vi "HFRR ADV v030 new software.vi"() -> ()   [LabVIEW 2025] (continued)
          frame #2 {
            n1890 = disable-structure shown="Disabled" {
              frame Disabled {
                w2654 = "cmd.exe  /c \"C:\\LAB-IQ-NXT\\UNOCOMPILE.bat\"" ("string")
                n1891 = local write "Prog Uno"(FALSE ("run minimized? (F)")) -> ()
                n1892 = call <vilib>:"System Exec.vi"("expected output size  (4096)"=u32 65535, "run minimized? (F)"=FALSE, "wait until completion? (T)"=TRUE ("run minimized? (F)"), "working directory"=path "C:/LAB-IQ-NXT", "standard input"=w2654, "command line"=w2654) -> ("error out"=w2653:errorcluster, "standard output"=→"String 42":string)  [unwired: 2 in, 2 out]
                "error out 3" <- w2653
                n1893 = flat-sequence {
                  tunnel: w2653 -> [_]
                  frame #0 {
                  }
                }
              }
              frame Enabled {
              }
            }
          }
        }
      }
    }
    n1894 = case shown="\"ISO 12156\"" "TEST STANDARD" {
      frame "ASTM D6079", Default {
        w2623 = 50.0 ("Hz")
        w2624 = 53.0 ("Set Rh")
        w2626 = 1.0 ("Set Strk")
        w2625 = 60.0 ("Set Temp")
        # "astm hide"
        n1895 = local write "NORMAL LOAD"(200.0 ("NORMAL LOAD")) -> ()
        n1896 = local write "Set Strk"(w2626) -> ()
        n1897 = local write "Set Hz"(w2623) -> ()
        n1898 = local write "Set Temp"(w2625) -> ()
        n1899 = local write "Set Rh"(w2624) -> ()
        n1900 = local write "test time"(75.0 ("test time")) -> ()
        n1901 = local write "Set Stroke:"(w2626) -> ()
        n1902 = local write "Set Humidity:"(w2624) -> ()
        n1903 = local write "Set Frequency:"(w2623) -> ()
        n1904 = local write "Set Temperature:"(w2625) -> ()
        "Test Standard" <- "ASTM D6079" ("Test Standard 2")
      }
      frame "ISO 12156" {
        n1905 = local write "Set Strk"(1.0 ("Set Strk")) -> ()
        n1906 = local write "NORMAL LOAD"(200.0 ("NORMAL LOAD")) -> ()
        n1907 = local write "Set Temp"(60.0 ("Set Temp")) -> ()
        n1908 = local write "test time"(75.0 ("test time")) -> ()
        n1909 = local write "Set Hz"(50.0 ("Hz")) -> ()
        n1910 = local write "Set Rh"(53.0 ("Set Rh")) -> ()
      }
      frame "CEC F-096-A-06" {
        n1911 = local write "Set Strk"(1.0 ("Set Strk")) -> ()
        n1912 = local write "NORMAL LOAD"(200.0 ("NORMAL LOAD")) -> ()
        n1913 = local write "Set Temp"(60.0 ("Set Temp")) -> ()
        n1914 = local write "test time"(75.0 ("test time")) -> ()
        n1915 = local write "Set Hz"(50.0 ("Hz")) -> ()
        n1916 = local write "Set Rh"(53.0 ("Set Rh")) -> ()
      }
      frame "Custom" {
      }
    }
    n1917 = Or(x=w2176, y=w2174) -> (x .or. y?=w2175:bool)
    n1918 = case shown="\"About\"" w2173 {
      tunnel: [T27."Acquire" ("Main Tab") T27."Compare Files" ("Main Tab") T27."About" ("Main Tab")] -> w2184
      frame "Acquire", Default {
      }
      frame "Compare Files" {
      }
      frame "About" {
      }
    }
    n1919 = Or(x=w2179, y="OPEN") -> (x .or. y?=w2180:bool)
    n1920 = case shown="True" w2180 {
      tunnel: w2179 -> [_ w2212]
      frame False {
      }
      frame True {
        n1921 = stacked-sequence {
          tunnel: w2212 -> [_ w2279 _ _]
          frame #0 {
            w2228 = "  " ("String 6")
            n1922 = local write "OPEN"(FALSE ("open")) -> ()
            n1923 = local read "string1 2"() -> (w2216:string)
            n1924 = local read "string1 3"() -> (w2215:string)
            n1925 = local read "string1 4"() -> (w2214:string)
            n1926 = property on="OPEN" class="Bool (strict)"("Visible"=FALSE) -> ()  [unwired: 2 in, 2 out]
            n1927 = local write "String 6"(w2228) -> ()
            n1928 = local write "String 7"(w2228) -> ()
            n1929 = local write "String 8"(w2228) -> ()
            n1930 = local write "String 12"(w2228) -> ()
            n1931 = local read "OK Button 16"() -> (w2213:bool)
            n1932 = String To Path(string=w2216) -> (path=w2224:path)
            n1933 = String To Path(string=w2215) -> (path=w2223:path)
            n1934 = String To Path(string=w2214) -> (path=w2222:path)
            n1935 = case shown="True" w2213 {
              tunnel: [w2229 w2230] -> w2217
              frame False {
                n1936 = local read "string1"() -> (w2229:string)
              }
              frame True {
                n1937 = local read "String Indicator 4"() -> (w2230:string)
              }
            }
            n1938 = Open/Create/Replace File "Open File"(file path (use dialog)=w2224) -> (refnum out=w2220:refnum<file>)  [unwired: 5 in, 2 out]
            n1939 = Open/Create/Replace File "Open File"(file path (use dialog)=w2223) -> (refnum out=w2219:refnum<file>)  [unwired: 5 in, 2 out]
            n1940 = Open/Create/Replace File "Open File"(file path (use dialog)=w2222) -> (refnum out=w2218:refnum<file>)  [unwired: 5 in, 2 out]
            n1941 = while {
              tunnel: w2220 -> [w2242]
              i -> [w2238]
              stop <- w2237 continue-if-true
              (unwired) TRUE ("line mode (F)")
              n1942 = Read from Text File "Read File"(file (use dialog)=w2242) -> (text=w2239:string)  [unwired: 3 in, 3 out]
              n1943 = local write "Numeric 11"(w2238) -> ()
              n1944 = String Length(string=w2239) -> (length=w2241:i32)
              n1945 = Greater?(x=w2241, y=1) -> (0:w2237:bool)
            }
            n1946 = while {
              tunnel: w2219 -> [w2248]
              i -> [w2244]
              stop <- w2243 continue-if-true
              (unwired) TRUE ("line mode (F)")
              n1947 = Read from Text File "Read File"(file (use dialog)=w2248) -> (text=w2245:string)  [unwired: 3 in, 3 out]
              n1948 = local write "Numeric 12"(w2244) -> ()
              n1949 = String Length(string=w2245) -> (length=w2247:i32)
              n1950 = Greater?(x=w2247, y=1) -> (0:w2243:bool)
            }
            n1951 = while {
              tunnel: w2218 -> [w2254]
              i -> [w2250]
              stop <- w2249 continue-if-true
              (unwired) TRUE ("line mode (F)")
              n1952 = Read from Text File "Read File"(file (use dialog)=w2254) -> (text=w2251:string)  [unwired: 3 in, 3 out]
              n1953 = local write "Numeric 13"(w2250) -> ()
              n1954 = String Length(string=w2251) -> (length=w2253:i32)
              n1955 = Greater?(x=w2253, y=1) -> (0:w2249:bool)
            }
            n1956 = String To Path(string=w2217) -> (path=w2225:path)
            n1957 = Open/Create/Replace File "Open File"(file path (use dialog)=w2225) -> (refnum out=w2221:refnum<file>)  [unwired: 5 in, 2 out]
            n1958 = while {
              tunnel: w2221 -> [w2236]
              i -> [w2232]
              stop <- w2231 continue-if-true
              (unwired) TRUE ("line mode (F)")
              n1959 = Read from Text File "Read File"(file (use dialog)=w2236) -> (text=w2233:string)  [unwired: 3 in, 3 out]
              n1960 = local write "Numeric 8"(w2232) -> ()
              n1961 = String Length(string=w2233) -> (length=w2235:i32)
              n1962 = Greater?(x=w2235, y=1) -> (0:w2231:bool)
            }
          }
          frame #1 {
            w2406 = FALSE ("ACTUAL   MERGE")
            # "Sample Temp"
            # "ECR"
            # "COF"
            # "Time\nCOF\nFF\nTemp"
            n1963 = case shown="True" w2279 {
              tunnel: [w2426 w2427] -> w2280
              frame False {
                n1964 = local read "string1"() -> (w2426:string)
              }
              frame True {
                n1965 = local read "String Indicator 4"() -> (w2427:string)
              }
            }
            n1966 = local read "string1 3"() -> (w2324:string)
            n1967 = String To Path(string=w2280) -> (path=w2411:path)
            n1968 = String To Path(string=w2324) -> (path=w2422:path)
            n1969 = local read "Numeric 12"() -> (w2408:i32)
            n1970 = local read "Numeric 8"() -> (w2410:i32)
            n1971 = local read "string1 2"() -> (w2325:string)
            n1972 = local read "string1 4"() -> (w2323:string)
            n1973 = Open/Create/Replace File "Open File"(file path (use dialog)=w2411) -> (refnum out=w2425:refnum<file>, error out=w2424:errorcluster)  [unwired: 5 in, 1 out]
            n1974 = Open/Create/Replace File "Open File"(file path (use dialog)=w2422) -> (refnum out=w2418:refnum<file>, error out=w2419:errorcluster)  [unwired: 5 in, 1 out]
            n1975 = for {
              N: w2410 -> [_]
              tunnel: w2425 -> [w2573]
              tunnel: w2424 -> [w2572]
              tunnel: [w2562] -> w2337 mode=indexing
              tunnel: [w2560] -> w2394 mode=indexing
              tunnel: [w2561] -> w2389 mode=indexing
              tunnel: w2406 -> [_]
              tunnel: [w2554] -> w2391 mode=indexing
              tunnel: [w2550] -> w2360 mode=indexing
              tunnel: [w2546] -> w2335 mode=indexing
              tunnel: [w2542] -> w2316 mode=indexing
              tunnel: [w2537] -> w2276 mode=indexing
              (unwired) TRUE ("line mode (F)")
              # "freq"
              # "Stroke"
              # "Time"
              # "CoF"
              # "Humidity"
              # "Temp"
              # "Air Temp"
              # "ECR"
              n1976 = Read from Text File "Read File"(file (use dialog)=w2573, error in=w2572) -> (text=w2538:string)  [unwired: 2 in, 3 out]
              n1977 = local write "String 6"(w2538) -> ()
              n1978 = String Subset(string=w2538, offset (0)=0, length (rest)=14 ("length (rest)")) -> (substring=w2566:string)
              n1979 = String Subset(string=w2538, offset (0)=35, length (rest)=9 ("length (rest)")) -> (substring=w2563:string)
              n1980 = String Subset(string=w2538, offset (0)=15, length (rest)=9 ("length (rest)")) -> (substring=w2569:string)
              n1981 = Fract/Exp String To Number(string=w2566) -> (number=w2562:dbl)  [unwired: 3 in, 1 out]
              n1982 = Fract/Exp String To Number(string=w2563) -> (number=w2561:dbl)  [unwired: 3 in, 1 out]
              n1983 = Fract/Exp String To Number(string=w2569) -> (number=w2560:dbl)  [unwired: 3 in, 1 out]
              n1984 = String Subset(string=w2538, offset (0)=85, length (rest)=9 ("length (rest)")) -> (substring=w2539:string)
              n1985 = String Subset(string=w2538, offset (0)=25, length (rest)=9 ("length (rest)")) -> (substring=w2545:string)
              n1986 = String Subset(string=w2538, offset (0)=55, length (rest)=9 ("length (rest)")) -> (substring=w2547:string)
              n1987 = String Subset(string=w2538, offset (0)=45, length (rest)=9 ("length (rest)")) -> (substring=w2553:string)
              n1988 = String Subset(string=w2538, offset (0)=65, length (rest)=9 ("length (rest)")) -> (substring=w2559:string)
              n1989 = Fract/Exp String To Number(string=w2545) -> (number=w2542:dbl)  [unwired: 3 in, 1 out]
              n1990 = Fract/Exp String To Number(string=w2539) -> (number=w2537:dbl)  [unwired: 3 in, 1 out]
              n1991 = Fract/Exp String To Number(string=w2547) -> (number=w2546:dbl)  [unwired: 3 in, 1 out]
              n1992 = Fract/Exp String To Number(string=w2553) -> (number=w2550:dbl)  [unwired: 3 in, 1 out]
              n1993 = Fract/Exp String To Number(string=w2559) -> (number=w2556:dbl)  [unwired: 3 in, 1 out]
              n1994 = Add(x=w2556, y=0.0) -> (x+y=w2554:dbl)
            }
            n1995 = for {
              N: w2408 -> [_]
              tunnel: w2419 -> [w2499]
              tunnel: w2418 -> [w2498]
              tunnel: [w2488] -> w2377 mode=indexing
              tunnel: [w2486] -> w2375 mode=indexing
              tunnel: [w2487] -> w2371 mode=indexing
              tunnel: w2406 -> [_]
              tunnel: [w2480] -> w2373 mode=indexing
              tunnel: [w2476] -> w2355 mode=indexing
              tunnel: [w2472] -> w2331 mode=indexing
              tunnel: [w2469] -> w2312 mode=indexing
              tunnel: [w2465] -> w2271 mode=indexing
              (unwired) 9 ("length (rest)")
              (unwired) 9 ("length (rest)")
              (unwired) TRUE ("line mode (F)")
              n1996 = Read from Text File "Read File"(file (use dialog)=w2498, error in=w2499) -> (text=w2466:string)  [unwired: 2 in, 3 out]
              n1997 = local write "String 8"(w2466) -> ()
              n1998 = String Subset(string=w2466, offset (0)=85) -> (substring=w2468:string)  [unwired: 1 in]
              n1999 = String Subset(string=w2466, offset (0)=35, length (rest)=9 ("length (rest)")) -> (substring=w2489:string)
              n2000 = String Subset(string=w2466, offset (0)=55, length (rest)=9 ("length (rest)")) -> (substring=w2474:string)
              n2001 = String Subset(string=w2466, offset (0)=25) -> (substring=w2470:string)  [unwired: 1 in]
              n2002 = String Subset(string=w2466, offset (0)=15, length (rest)=9 ("length (rest)")) -> (substring=w2495:string)
              n2003 = String Subset(string=w2466, offset (0)=0, length (rest)=14 ("length (rest)")) -> (substring=w2492:string)
              n2004 = String Subset(string=w2466, offset (0)=45, length (rest)=9 ("length (rest)")) -> (substring=w2479:string)
              n2005 = String Subset(string=w2466, offset (0)=65, length (rest)=9 ("length (rest)")) -> (substring=w2485:string)
              n2006 = Fract/Exp String To Number(string=w2468) -> (number=w2465:dbl)  [unwired: 3 in, 1 out]
              n2007 = Fract/Exp String To Number(string=w2489) -> (number=w2487:dbl)  [unwired: 3 in, 1 out]
              n2008 = Fract/Exp String To Number(string=w2474) -> (number=w2472:dbl)  [unwired: 3 in, 1 out]
              n2009 = Fract/Exp String To Number(string=w2470) -> (number=w2469:dbl)  [unwired: 3 in, 1 out]
              n2010 = Fract/Exp String To Number(string=w2495) -> (number=w2486:dbl)  [unwired: 3 in, 1 out]
              n2011 = Fract/Exp String To Number(string=w2492) -> (number=w2488:dbl)  [unwired: 3 in, 1 out]
              n2012 = Fract/Exp String To Number(string=w2479) -> (number=w2476:dbl)  [unwired: 3 in, 1 out]
              n2013 = Fract/Exp String To Number(string=w2485) -> (number=w2482:dbl)  [unwired: 3 in, 1 out]
              n2014 = Add(x=w2482, y=0.0) -> (x+y=w2480:dbl)
            }
            n2015 = String To Path(string=w2325) -> (path=w2423:path)
            n2016 = String To Path(string=w2323) -> (path=w2417:path)
            n2017 = local read "Numeric 11"() -> (w2407:i32)
            n2018 = local read "Numeric 13"() -> (w2409:i32)
            n2019 = Open/Create/Replace File "Open File"(file path (use dialog)=w2423) -> (refnum out=w2421:refnum<file>, error out=w2420:errorcluster)  [unwired: 5 in, 1 out]
            n2020 = Open/Create/Replace File "Open File"(file path (use dialog)=w2417) -> (refnum out=w2416:refnum<file>, error out=w2415:errorcluster)  [unwired: 5 in, 1 out]
            n2021 = for {
              N: w2407 -> [_]
              tunnel: w2421 -> [w2536]
              tunnel: w2420 -> [w2535]
              tunnel: [w2525] -> w2387 mode=indexing
              tunnel: [w2523] -> w2385 mode=indexing
              tunnel: [w2524] -> w2380 mode=indexing
              tunnel: w2406 -> [_]
              tunnel: [w2517] -> w2382 mode=indexing
              tunnel: [w2513] -> w2358 mode=indexing
              tunnel: [w2509] -> w2333 mode=indexing
              tunnel: [w2505] -> w2314 mode=indexing
              tunnel: [w2500] -> w2272 mode=indexing
              (unwired) TRUE ("line mode (F)")
              n2022 = Read from Text File "Read File"(file (use dialog)=w2536, error in=w2535) -> (text=w2501:string)  [unwired: 2 in, 3 out]
              n2023 = local write "String 7"(w2501) -> ()
              n2024 = String Subset(string=w2501, offset (0)=85, length (rest)=9 ("length (rest)")) -> (substring=w2504:string)
              n2025 = String Subset(string=w2501, offset (0)=35, length (rest)=9 ("length (rest)")) -> (substring=w2526:string)
              n2026 = String Subset(string=w2501, offset (0)=55, length (rest)=9 ("length (rest)")) -> (substring=w2512:string)
              n2027 = String Subset(string=w2501, offset (0)=25, length (rest)=9 ("length (rest)")) -> (substring=w2506:string)
              n2028 = String Subset(string=w2501, offset (0)=45, length (rest)=9 ("length (rest)")) -> (substring=w2514:string)
              n2029 = String Subset(string=w2501, offset (0)=0, length (rest)=14 ("length (rest)")) -> (substring=w2529:string)
              n2030 = String Subset(string=w2501, offset (0)=15, length (rest)=9 ("length (rest)")) -> (substring=w2532:string)
              n2031 = String Subset(string=w2501, offset (0)=65, length (rest)=9 ("length (rest)")) -> (substring=w2518:string)
              n2032 = Fract/Exp String To Number(string=w2504) -> (number=w2500:dbl)  [unwired: 3 in, 1 out]
              n2033 = Fract/Exp String To Number(string=w2526) -> (number=w2524:dbl)  [unwired: 3 in, 1 out]
              n2034 = Fract/Exp String To Number(string=w2512) -> (number=w2509:dbl)  [unwired: 3 in, 1 out]
              n2035 = Fract/Exp String To Number(string=w2506) -> (number=w2505:dbl)  [unwired: 3 in, 1 out]
              n2036 = Fract/Exp String To Number(string=w2514) -> (number=w2513:dbl)  [unwired: 3 in, 1 out]
              n2037 = Fract/Exp String To Number(string=w2529) -> (number=w2525:dbl)  [unwired: 3 in, 1 out]
              n2038 = Fract/Exp String To Number(string=w2532) -> (number=w2523:dbl)  [unwired: 3 in, 1 out]
              n2039 = Fract/Exp String To Number(string=w2518) -> (number=w2521:dbl)  [unwired: 3 in, 1 out]
              n2040 = Add(x=w2521, y=0.0) -> (x+y=w2517:dbl)
            }
            n2041 = for {
              N: w2409 -> [_]
              tunnel: w2416 -> [w2464]
              tunnel: w2415 -> [w2463]
              tunnel: [w2453] -> w2369 mode=indexing
              tunnel: [w2452] -> w2362 mode=indexing
              tunnel: w2406 -> [_]
              tunnel: [w2441] -> w2367 mode=indexing
              tunnel: [w2446] -> w2364 mode=indexing
              tunnel: [w2442] -> w2354 mode=indexing
              tunnel: [w2437] -> w2329 mode=indexing
              tunnel: [w2433] -> w2310 mode=indexing
              tunnel: [w2428] -> w2270 mode=indexing
              (unwired) 1.0 ("x")
              (unwired) TRUE ("line mode (F)")
              n2042 = Read from Text File "Read File"(file (use dialog)=w2464, error in=w2463) -> (text=w2429:string)  [unwired: 2 in, 3 out]
              n2043 = local write "String 12"(w2429) -> ()
              n2044 = String Subset(string=w2429, offset (0)=85, length (rest)=9 ("length (rest)")) -> (substring=w2431:string)
              n2045 = String Subset(string=w2429, offset (0)=35, length (rest)=9 ("length (rest)")) -> (substring=w2454:string)
              n2046 = String Subset(string=w2429, offset (0)=55, length (rest)=9 ("length (rest)")) -> (substring=w2439:string)
              n2047 = String Subset(string=w2429, offset (0)=25, length (rest)=9 ("length (rest)")) -> (substring=w2435:string)
              n2048 = String Subset(string=w2429, offset (0)=45, length (rest)=9 ("length (rest)")) -> (substring=w2444:string)
              n2049 = String Subset(string=w2429, offset (0)=15, length (rest)=9 ("length (rest)")) -> (substring=w2460:string)
              n2050 = String Subset(string=w2429, offset (0)=0, length (rest)=14 ("length (rest)")) -> (substring=w2457:string)
              n2051 = String Subset(string=w2429, offset (0)=65, length (rest)=9 ("length (rest)")) -> (substring=w2447:string)
              n2052 = Fract/Exp String To Number(string=w2431) -> (number=w2428:dbl)  [unwired: 3 in, 1 out]
              n2053 = Fract/Exp String To Number(string=w2454) -> (number=w2452:dbl)  [unwired: 3 in, 1 out]
              n2054 = Fract/Exp String To Number(string=w2439) -> (number=w2437:dbl)  [unwired: 3 in, 1 out]
              n2055 = Fract/Exp String To Number(string=w2435) -> (number=w2433:dbl)  [unwired: 3 in, 1 out]
              n2056 = Fract/Exp String To Number(string=w2444) -> (number=w2442:dbl)  [unwired: 3 in, 1 out]
              n2057 = Fract/Exp String To Number(string=w2460) -> (number=w2441:dbl)  [unwired: 3 in, 1 out]
              n2058 = Fract/Exp String To Number(string=w2457) -> (number=w2453:dbl)  [unwired: 3 in, 1 out]
              n2059 = Fract/Exp String To Number(string=w2447) -> (number=w2450:dbl)  [unwired: 3 in, 1 out]
              n2060 = Add(x=w2450, y=0.0) -> (x+y=w2446:dbl)
            }
            n2061 = Delete From Array(array=w2312, index=0) -> (array with subset deleted=w2285:dbl[])  [unwired: 1 in, 1 out]
            n2062 = Delete From Array(array=w2375, index=0) -> (array with subset deleted=w2348:dbl[])  [unwired: 1 in, 1 out]
            n2063 = Delete From Array(array=w2355, index=0) -> (array with subset deleted=w2343:dbl[])  [unwired: 1 in, 1 out]
            n2064 = Delete From Array(array=w2373, index=0) -> (array with subset deleted=w2374:dbl[])  [unwired: 1 in, 1 out]
            n2065 = call-poly <vilib>:"Mean.vi"("X"=w2285) -> ("mean"=→"КОФ2 4":dbl)  [unwired: 1 out]
            n2066 = call-poly <vilib>:"Mean.vi"("X"=w2348) -> ("mean"=→"КОФ3":dbl)  [unwired: 1 out]
            n2067 = call-poly <vilib>:"Mean.vi"("X"=w2343) -> ("mean"=→"CP3":dbl)  [unwired: 1 out]
            n2068 = Delete From Array(array=w2337, index=0) -> (array with subset deleted=w2264:dbl[])  [unwired: 1 in, 1 out]
            n2069 = Delete From Array(array=w2276, index=0) -> (array with subset deleted=w2263:dbl[])  [unwired: 1 in, 1 out]
            n2070 = Delete From Array(array=w2316, index=0) -> (array with subset deleted=w2287:dbl[])  [unwired: 1 in, 1 out]
            n2071 = Delete From Array(array=w2394, index=0) -> (array with subset deleted=w2349:dbl[])  [unwired: 1 in, 1 out]
            n2072 = Delete From Array(array=w2360, index=0) -> (array with subset deleted=w2345:dbl[])  [unwired: 1 in, 1 out]
            "array w/ subset deleted" <- w2345
            n2073 = Delete From Array(array=w2391, index=0) -> (array with subset deleted=w2392:dbl[])  [unwired: 1 in, 1 out]
            n2074 = call-poly <vilib>:"Mean.vi"("X"=w2287) -> ("mean"=→"КОФ2 2":dbl)  [unwired: 1 out]
            n2075 = call-poly <vilib>:"Mean.vi"("X"=w2349) -> ("mean"=→"КОФ1":dbl)  [unwired: 1 out]
            n2076 = Bundle "Bundle"(w2264, w2263) -> (w2269:cluster{dbl[], dbl[]})  [unwired: 1 in]
            n2077 = Bundle "Bundle"(w2264, w2392) -> (w2256:cluster{dbl[], dbl[]})  [unwired: 1 in]
            n2078 = Delete From Array(array=w2271, index=0) -> (array with subset deleted=w2259:dbl[])  [unwired: 1 in, 1 out]
            n2079 = Delete From Array(array=w2272, index=0) -> (array with subset deleted=w2261:dbl[])  [unwired: 1 in, 1 out]
            n2080 = Delete From Array(array=w2382, index=0) -> (array with subset deleted=w2383:dbl[])  [unwired: 1 in, 1 out]
            n2081 = Delete From Array(array=w2270, index=0) -> (array with subset deleted=w2257:dbl[])  [unwired: 1 in, 1 out]
            n2082 = Delete From Array(array=w2364, index=0) -> (array with subset deleted=w2365:dbl[])  [unwired: 1 in, 1 out]
            n2083 = Delete From Array(array=w2389, index=0) -> (array with subset deleted=w2295:dbl[])  [unwired: 1 in, 1 out]
            n2084 = Delete From Array(array=w2335, index=0) -> (array with subset deleted=w2291:dbl[])  [unwired: 1 in, 1 out]
            n2085 = Delete From Array(array=w2371, index=0) -> (array with subset deleted=w2293:dbl[])  [unwired: 1 in, 1 out]
            n2086 = Delete From Array(array=w2331, index=0) -> (array with subset deleted=w2289:dbl[])  [unwired: 1 in, 1 out]
            n2087 = Delete From Array(array=w2380, index=0) -> (array with subset deleted=w2294:dbl[])  [unwired: 1 in, 1 out]
            n2088 = Delete From Array(array=w2333, index=0) -> (array with subset deleted=w2290:dbl[])  [unwired: 1 in, 1 out]
            n2089 = Delete From Array(array=w2314, index=0) -> (array with subset deleted=w2286:dbl[])  [unwired: 1 in, 1 out]
            n2090 = Delete From Array(array=w2358, index=0) -> (array with subset deleted=w2344:dbl[])  [unwired: 1 in, 1 out]
            n2091 = Delete From Array(array=w2385, index=0) -> (array with subset deleted=w2346:dbl[])  [unwired: 1 in, 1 out]
            n2092 = Delete From Array(array=w2362, index=0) -> (array with subset deleted=w2292:dbl[])  [unwired: 1 in, 1 out]
            n2093 = Delete From Array(array=w2329, index=0) -> (array with subset deleted=w2288:dbl[])  [unwired: 1 in, 1 out]
            n2094 = Delete From Array(array=w2310, index=0) -> (array with subset deleted=w2284:dbl[])  [unwired: 1 in, 1 out]
            n2095 = Delete From Array(array=w2354, index=0) -> (array with subset deleted=w2342:dbl[])  [unwired: 1 in, 1 out]
            n2096 = Delete From Array(array=w2367, index=0) -> (array with subset deleted=w2347:dbl[])  [unwired: 1 in, 1 out]
            n2097 = Delete From Array(array=w2377, index=0) -> (array with subset deleted=w2260:dbl[])  [unwired: 1 in, 1 out]
            n2098 = Delete From Array(array=w2387, index=0) -> (array with subset deleted=w2262:dbl[])  [unwired: 1 in, 1 out]
            n2099 = Delete From Array(array=w2369, index=0) -> (array with subset deleted=w2258:dbl[])  [unwired: 1 in, 1 out]
            n2100 = Bundle "Bundle"(w2264, w2295) -> (w2282:cluster{dbl[], dbl[]})  [unwired: 1 in]
            n2101 = Bundle "Bundle"(w2264, w2349) -> (w2283:cluster{dbl[], dbl[]})  [unwired: 1 in]
            n2102 = Bundle "Bundle"(w2295, w2291) -> (w2297:cluster{dbl[], dbl[]})  [unwired: 1 in]
            n2103 = Bundle "Bundle"(w2260, w2259) -> (w2267:cluster{dbl[], dbl[]})  [unwired: 1 in]
            n2104 = Bundle "Bundle"(w2293, w2289) -> (w2299:cluster{dbl[], dbl[]})  [unwired: 1 in]
            n2105 = Bundle "Bundle"(w2260, w2293) -> (w2403:cluster{dbl[], dbl[]})  [unwired: 1 in]
            n2106 = Bundle "Bundle"(w2260, w2289) -> (w2327:cluster{dbl[], dbl[]})  [unwired: 1 in]
            n2107 = Bundle "Bundle"(w2260, w2348) -> (w2413:cluster{dbl[], dbl[]})  [unwired: 1 in]
            n2108 = Bundle "Bundle"(w2260, w2343) -> (w2351:cluster{dbl[], dbl[]})  [unwired: 1 in]
            n2109 = Bundle "Bundle"(w2260, w2374) -> (w2398:cluster{dbl[], dbl[]})  [unwired: 1 in]
            n2110 = Bundle "Bundle"(w2294, w2290) -> (w2298:cluster{dbl[], dbl[]})  [unwired: 1 in]
            n2111 = Bundle "Bundle"(w2262, w2261) -> (w2268:cluster{dbl[], dbl[]})  [unwired: 1 in]
            n2112 = Bundle "Bundle"(w2262, w2294) -> (w2405:cluster{dbl[], dbl[]})  [unwired: 1 in]
            n2113 = Bundle "Bundle"(w2262, w2290) -> (w2328:cluster{dbl[], dbl[]})  [unwired: 1 in]
            n2114 = Bundle "Bundle"(w2262, w2344) -> (w2352:cluster{dbl[], dbl[]})  [unwired: 1 in]
            n2115 = Bundle "Bundle"(w2262, w2346) -> (w2414:cluster{dbl[], dbl[]})  [unwired: 1 in]
            n2116 = Bundle "Bundle"(w2262, w2383) -> (w2396:cluster{dbl[], dbl[]})  [unwired: 1 in]
            n2117 = Bundle "Bundle"(w2292, w2288) -> (w2300:cluster{dbl[], dbl[]})  [unwired: 1 in]
            n2118 = Bundle "Bundle"(w2258, w2257) -> (w2266:cluster{dbl[], dbl[]})  [unwired: 1 in]
            n2119 = Bundle "Bundle"(w2258, w2292) -> (w2404:cluster{dbl[], dbl[]})  [unwired: 1 in]
            n2120 = Bundle "Bundle"(w2258, w2288) -> (w2326:cluster{dbl[], dbl[]})  [unwired: 1 in]
            n2121 = Bundle "Bundle"(w2258, w2342) -> (w2350:cluster{dbl[], dbl[]})  [unwired: 1 in]
            n2122 = Bundle "Bundle"(w2258, w2347) -> (w2412:cluster{dbl[], dbl[]})  [unwired: 1 in]
            n2123 = Bundle "Bundle"(w2258, w2365) -> (w2397:cluster{dbl[], dbl[]})  [unwired: 1 in]
            n2124 = call-poly <vilib>:"Mean.vi"("X"=w2345) -> ("mean"=→"CP1":dbl)  [unwired: 1 out]
            n2125 = call-poly <vilib>:"Mean.vi"("X"=w2286) -> ("mean"=→"КОФ2 3":dbl)  [unwired: 1 out]
            n2126 = call-poly <vilib>:"Mean.vi"("X"=w2344) -> ("mean"=→"CP2":dbl)  [unwired: 1 out]
            n2127 = call-poly <vilib>:"Mean.vi"("X"=w2346) -> ("mean"=→"КОФ2":dbl)  [unwired: 1 out]
            n2128 = call-poly <vilib>:"Mean.vi"("X"=w2284) -> ("mean"=→"КОФ2 5":dbl)  [unwired: 1 out]
            n2129 = call-poly <vilib>:"Mean.vi"("X"=w2342) -> ("mean"=→"CP4":dbl)  [unwired: 1 out]
            n2130 = call-poly <vilib>:"Mean.vi"("X"=w2347) -> ("mean"=→"КОФ4":dbl)  [unwired: 1 out]
            n2131 = Bundle "Bundle"(w2264, w2291) -> (w2255:cluster{dbl[], dbl[]})  [unwired: 1 in]
            n2132 = Bundle "Bundle"(w2264, w2345) -> (w2278:cluster{dbl[], dbl[]})  [unwired: 1 in]
            n2133 = Build Array "Build Array"(w2255, w2278) -> (w2281:cluster{dbl[], dbl[]}[])
            "XY Graph 17" <- w2281
            n2134 = Build Array "Build Array"(w2269, w2268, w2267, w2266) -> (→"Frequency ( Hz )":cluster{dbl[], dbl[]}[])
            n2135 = Build Array "Build Array"(w2297, w2298, w2299, w2300) -> (→"Air Temp ( °C ) vs Humidity ( % RH )":cluster{dbl[], dbl[]}[])
            n2136 = Build Array "Build Array"(w2282, w2405, w2403, w2404) -> (→"Air Temperature  ( °C )":cluster{dbl[], dbl[]}[])
            n2137 = Build Array "Build Array"(w2255, w2328, w2327, w2326) -> (→"Humidity ( %RH )":cluster{dbl[], dbl[]}[])
            n2138 = Build Array "Build Array"(w2283, w2414, w2413, w2412) -> (→"Coefficient Of Friction":cluster{dbl[], dbl[]}[])
            n2139 = Build Array "Build Array"(w2278, w2352, w2351, w2350) -> (→"Sample Temperature ( °C )":cluster{dbl[], dbl[]}[])
            n2140 = Build Array "Build Array"(w2256, w2396, w2398, w2397) -> (→"XY Graph 13":cluster{dbl[], dbl[]}[])
            n2141 = Bundle "Bundle"(w2264, w2287) -> (w2309:cluster{dbl[], dbl[]})  [unwired: 1 in]
            n2142 = Bundle "Bundle"(w2260, w2285) -> (w2307:cluster{dbl[], dbl[]})  [unwired: 1 in]
            n2143 = Bundle "Bundle"(w2262, w2286) -> (w2308:cluster{dbl[], dbl[]})  [unwired: 1 in]
            n2144 = Bundle "Bundle"(w2258, w2284) -> (w2306:cluster{dbl[], dbl[]})  [unwired: 1 in]
            n2145 = Build Array "Build Array"(w2309, w2308, w2307, w2306) -> (→"Stroke ( mm )":cluster{dbl[], dbl[]}[])
            n2146 = local write "XY Graph 16"(w2281) -> ()
          }
          frame #2 {
          }
          frame #3 {
            n2147 = local write "Numeric 8"(0 ("Numeric 8")) -> ()
            n2148 = local write "Numeric 11"(0 ("Numeric 11")) -> ()
            n2149 = local write "Numeric 12"(0 ("Numeric 12")) -> ()
            n2150 = local write "Numeric 13"(0 ("Numeric 13")) -> ()
            n2151 = property on="OPEN" class="Bool (strict)"("Visible"=TRUE) -> ()  [unwired: 2 in, 2 out]
            n2152 = local read "String Control 2"() -> (w2581:string)
            n2153 = local read "String Control 4"() -> (w2580:string)
            n2154 = local read "String Control 6"() -> (w2579:string)
            n2155 = local read "String Control 8"() -> (w2578:string)
            n2156 = Match Pattern(string=w2581, regular expression="Samples / cycle :- ") -> (after substring=w2595:string)  [unwired: 1 in, 3 out]
            n2157 = Match Pattern(string=w2581, regular expression="Frequency :- ") -> (after substring=w2614:string)  [unwired: 1 in, 3 out]
            n2158 = Match Pattern(string=w2580, regular expression="Samples / cycle :- ") -> (after substring=w2591:string)  [unwired: 1 in, 3 out]
            n2159 = Match Pattern(string=w2580, regular expression="Frequency :- ") -> (after substring=w2609:string)  [unwired: 1 in, 3 out]
            n2160 = Match Pattern(string=w2579, regular expression="Samples / cycle :- ") -> (after substring=w2587:string)  [unwired: 1 in, 3 out]
            n2161 = Match Pattern(string=w2579, regular expression="Frequency :- ") -> (after substring=w2604:string)  [unwired: 1 in, 3 out]
            n2162 = Match Pattern(string=w2578, regular expression="Samples / cycle :- ") -> (after substring=w2583:string)  [unwired: 1 in, 3 out]
            n2163 = Match Pattern(string=w2578, regular expression="Frequency :- ") -> (after substring=w2599:string)  [unwired: 1 in, 3 out]
            n2164 = String Subset(string=w2595, length (rest)=6 ("length (rest)")) -> (substring=w2597:string)  [unwired: 1 in]
            n2165 = String Subset(string=w2614, length (rest)=9 ("length (rest)")) -> (substring=w2616:string)  [unwired: 1 in]
            n2166 = String Subset(string=w2591, length (rest)=6 ("length (rest)")) -> (substring=w2593:string)  [unwired: 1 in]
            n2167 = String Subset(string=w2609, length (rest)=9 ("length (rest)")) -> (substring=w2611:string)  [unwired: 1 in]
            n2168 = String Subset(string=w2587, length (rest)=6 ("length (rest)")) -> (substring=w2589:string)  [unwired: 1 in]
            n2169 = String Subset(string=w2604, length (rest)=9 ("length (rest)")) -> (substring=w2606:string)  [unwired: 1 in]
            n2170 = String Subset(string=w2583, length (rest)=6 ("length (rest)")) -> (substring=w2585:string)  [unwired: 1 in]
            n2171 = String Subset(string=w2599, length (rest)=9 ("length (rest)")) -> (substring=w2601:string)  [unwired: 1 in]
            n2172 = Fract/Exp String To Number(string=w2597) -> (number=w2577:dbl)  [unwired: 3 in, 1 out]
            n2173 = Fract/Exp String To Number(string=w2616) -> (number=w2617:dbl)  [unwired: 3 in, 1 out]
            n2174 = Fract/Exp String To Number(string=w2593) -> (number=w2576:dbl)  [unwired: 3 in, 1 out]
            n2175 = Fract/Exp String To Number(string=w2611) -> (number=w2612:dbl)  [unwired: 3 in, 1 out]
            n2176 = Fract/Exp String To Number(string=w2589) -> (number=w2575:dbl)  [unwired: 3 in, 1 out]
            n2177 = Fract/Exp String To Number(string=w2606) -> (number=w2607:dbl)  [unwired: 3 in, 1 out]
            n2178 = Fract/Exp String To Number(string=w2585) -> (number=w2574:dbl)  [unwired: 3 in, 1 out]
            n2179 = Fract/Exp String To Number(string=w2601) -> (number=w2602:dbl)  [unwired: 3 in, 1 out]
            n2180 = local write "sample1"(w2577) -> ()
            n2181 = local write "freq1"(w2617) -> ()
            n2182 = local write "sample2"(w2576) -> ()
            n2183 = local write "freq2"(w2612) -> ()
            n2184 = local write "sample3"(w2575) -> ()
            n2185 = local write "freq3"(w2607) -> ()
            n2186 = local write "sample4"(w2574) -> ()
            n2187 = local write "freq 4"(w2602) -> ()
          }
        }
      }
    }
    n2188 = case shown="True" w2175 {
      selector: w2175 -> [_ w2194]
      frame False {
      }
      frame True {
        n2189 = Not(x=w2194) -> (.not. x?=w2190:bool)
        n2190 = local write "service 3"(w2190) -> ()
        n2191 = local write "OPEN 6"(w2190) -> ()
        n2192 = call <vilib>:"System Exec.vi"("wait until completion? (T)"=TRUE, "command line"="C:\\LAB-IQ\\Scar View.exe") -> ("error out"=→"error out 5":errorcluster)  [unwired: 6 in, 3 out]
      }
    }
    n2193 = case shown="\"Acquire\", Default" w2184 {
      frame "Acquire", Default {
        # "Elapsed time\ncof\nstroke\nAir temp\nTemp\nHumidity"
        n2194 = disable-structure shown="Disabled" {
          frame Disabled {
            n2195 = local read "Flag"() -> (w2893:dbl)
            n2196 = local read "RUN"() -> (w2890:bool)
            n2197 = Not(x=w2890) -> (.not. x?=w2889:bool)
            n2198 = Equal?(x=w2893, y=10.0) -> (x = y?=w2891:bool)
            n2199 = And(x=w2891, y=w2889) -> (x .and. y?=w2888:bool)
            n2200 = case shown="True" w2888 {
              frame False {
              }
              frame True {
                w2894 = FALSE ("Heater Button")
                n2201 = local write "Humidity"(w2894) -> ()
                n2202 = local write "Heater Button"(w2894) -> ()
              }
            }
          }
          frame Enabled {
          }
        }
        n2203 = disable-structure shown="Disabled" {
          frame Disabled {
            n2204 = case shown="True" {
              selector: _ -> [_ _]
              frame False {
              }
              frame True {
                w2947 = TRUE ("Heater")
                n2205 = local write "Humidity"(w2947) -> ()
                n2206 = local write "Heater Button"(w2947) -> ()
                n2207 = local read "TEST STANDARD"() -> (w2950:T3)
                n2208 = local read "TEST STANDARD"() -> (w2945:T3)
                n2209 = Equal?(x=w2950, y=enum16{"ASTM D6079", "ISO 12156", "Custom"}."ISO 12156" ("Test Standard")) -> (x = y?=w2948:bool)
                n2210 = Equal?(x=w2945, y=enum16{"ASTM D6079", "ISO 12156", "Custom"}."ASTM D6079" ("Test Standard")) -> (x = y?=w2944:bool)
                n2211 = case shown="True" w2948 {
                  frame False {
                  }
                  frame True {
                    n2212 = local write "airtempflg"(FALSE ("airtempflg")) -> ()
                    n2213 = local write item#-1(TRUE ("Heater")) -> ()
                  }
                }
                n2214 = case shown="True" w2944 {
                  frame False {
                  }
                  frame True {
                    n2215 = local write "airtempflg"(TRUE ("airtempflg")) -> ()
                    n2216 = local write item#-1(FALSE ("Heater")) -> ()
                  }
                }
              }
            }
          }
          frame Enabled {
          }
        }
        n2217 = stacked-sequence {
          frame #0 {
            n2218 = case shown="True" "RST FF" {
              frame False {
              }
              frame True {
                w2964 = 0.0 ("X Scale.Range:Maximum")
                n2219 = property on="Frictional Force ( N )" class="WFChart (strict)"("XScale.Maximum"=600.0 ("X Scale.Range:Maximum"), "XScale.Minimum"=w2964, "YScale.Maximum"=10.0 ("Y Scale.Range:Maximum"), "YScale.Minimum"=w2964) -> ()  [unwired: 2 in, 2 out]
              }
            }
          }
          frame #1 {
            n2220 = case shown="True" "RST TEMP" {
              frame False {
              }
              frame True {
                n2221 = property on="Temperature ( Deg C )" class="WFChart (strict)"("XScale.Minimum"=0.0 ("X Scale.Range:Minimum"), "XScale.Maximum"=600.0 ("X Scale.Range:Maximum"), "YScale.Minimum"=0.0 ("Y Scale.Range:Minimum"), "YScale.Maximum"=100.0 ("Y Scale.Range:Maximum")) -> ()  [unwired: 2 in, 2 out]
              }
            }
          }
          frame #2 {
            n2222 = case shown="True" "RSTCOF" {
              frame False {
              }
              frame True {
                n2223 = property on="Coefficient of Friction" class="WFChart (strict)"("XScale.Minimum"=0.0 ("X Scale.Range:Minimum"), "XScale.Maximum"=600.0 ("X Scale.Range:Maximum"), "YScale.Maximum"=1.0 ("X Scale.Range:Minimum"), "YScale.Minimum"=0.0 ("X Scale.Range:Minimum")) -> ()  [unwired: 2 in, 2 out]
              }
            }
          }
          frame #3 {
            n2224 = case shown="True" "RSTCOF 2" {
              frame False {
              }
              frame True {
                (unwired) 100.0 ("Y Scale.Range:Maximum")
                (unwired) 0.0 ("Y Scale.Range:Minimum")
                (unwired) 600.0 ("X Scale.Range:Maximum")
                (unwired) 0.0 ("X Scale.Range:Minimum")
              }
            }
          }
          frame #4 {
            n2225 = case shown="True" "RSTCOF 3" {
              frame False {
              }
              frame True {
                n2226 = property on="Electrical Contact Resistance ( % )" class="WFChart (strict)"("XScale.Minimum"=0.0 ("X Scale.Range:Minimum"), "XScale.Maximum"=600.0 ("X Scale.Range:Maximum"), "YScale.Minimum"=0.0 ("Y Scale.Range:Minimum"), "YScale.Maximum"=100.0 ("Y Scale.Range:Maximum")) -> ()  [unwired: 2 in, 2 out]
              }
            }
          }
        }
        n2227 = local read "RUN"() -> (w2883:bool)
        n2228 = case shown="False" w2883 {
          frame False {
          }
          frame True {
          }
        }
        n2229 = local read "RUN"() -> (w2887:bool)
        n2230 = case shown="False" w2887 {
          tunnel: [FALSE ("TEST RUNNING") TRUE ("TEST RUNNING")] -> w2886
          frame False {
            w2983 = 0.0 ("Flag")
            n2231 = local write "Elapsed time"(0.0 ("elapsedtime")) -> ()
            n2232 = local write "Time Remaining"(w2983) -> ()
            n2233 = local write "Flag"(w2983) -> ()
            n2234 = local write "Remaining Time"(w2983) -> ()
          }
          frame True {
            n2235 = local write "Flag"(10.0 ("Flag")) -> ()
          }
        }
        n2236 = local read "AIR TEMP"() -> (w2881:dbl)
        n2237 = Greater Or Equal?(x=w2881, y=15.0) -> (x >= y?=w2882:bool)
        "powstat" <- w2882
        n2238 = case shown="True" "Save & Continue" {
          frame False {
          }
          frame True {
            n2239 = local read "USER ID"() -> (w3277:string)
            n2240 = local read "FILE"() -> (w3285:string)
            n2241 = String Length(string=w3285) -> (length=w3283:i32)
            n2242 = String Length(string=w3277) -> (length=w3280:i32)
            n2243 = Greater?(x=w3283, y=0) -> (0:w3282:bool)
            n2244 = Greater?(x=w3280, y=0) -> (0:w3279:bool)
            n2245 = And(x=w3282, y=w3279) -> (x .and. y?=w3278:bool)
            n2246 = case shown="True" w3278 {
              frame False {
                n2247 = stacked-sequence {
                  frame #0 {
                    n2248 = One Button Dialog(message="Please Enter a File Name and Operator ID to save data !", button name ("OK")="Ok") -> ()  [unwired: 1 out]
                  }
                  frame #1 {
                    n2249 = local write "Save & Continue"(FALSE ("OK Button")) -> ()
                  }
                }
                n2250 = local write "Save & Continue"(FALSE ("OK Button")) -> ()
              }
              frame True {
                n2251 = stacked-sequence {
                  frame #0 {
                    n2252 = local read "FILE"() -> (w3291:string)
                    n2253 = call "file check.vi"("file name in"=w3291) -> ("file name out"=w3290:string)  [unwired: 9 in, 1 out]
                    n2254 = call <vilib>:"Application Directory.vi"() -> ("Application Directory"=w3301:path)
                    n2255 = Build Path(base path=w3301, name or relative path="data") -> (appended path=w3300:path)
                    n2256 = call <vilib>:"Trim Whitespace.vi"("string"=w3290) -> ("trimmed string"=w3298:string)  [unwired: 1 in]
                    n2257 = call <vilib>:"Trim Whitespace.vi"("string"=w3290) -> ("trimmed string"=w3299:string)  [unwired: 1 in]
                    n2258 = List Folder(path=w3300) -> (folder names=w3296:string[])  [unwired: 3 in, 3 out]
                    n2259 = Match Pattern(string=w3298, regular expression="_(") -> (before substring=w3295:string)  [unwired: 1 in, 3 out]
                    n2260 = for {
                      tunnel: w3296 -> [w3310] mode=indexing
                      tunnel: w3295 -> [w3308]
                      shift-right: [w3306] -> w3293
                      shift-left: bool[] [] -> [w3307]
                      n2261 = Match Pattern(string=w3310, regular expression="_(") -> (before substring=w3309:string)  [unwired: 1 in, 3 out]
                      n2262 = Equal?(x=w3309, y=w3308) -> (x = y?=w3305:bool)
                      n2263 = case shown="True" w3305 {
                        tunnel: w3305 -> [_ w3313]
                        tunnel: w3307 -> [w3312 w3315]
                        tunnel: [w3312 w3314] -> w3306
                        frame False {
                        }
                        frame True {
                          n2264 = Insert Into Array(array=w3315, new element=w3313) -> (w3314:bool[])  [unwired: 1 in]
                        }
                      }
                    }
                    n2265 = Equal?(x=w3296, y=w3295) -> (x = y?=w3304:bool[])
                    n2266 = Or Array Elements(Boolean array=w3304) -> (logical OR=w3303:bool)
                    n2267 = Array Size(array=w3293) -> (size(s)=w3292:i32)
                    n2268 = case shown="True" w3303 {
                      tunnel: w3299 -> [_ w3323]
                      tunnel: w3292 -> [_ w3316]
                      frame False {
                      }
                      frame True {
                        n2269 = Number To Decimal String(number=w3316) -> (decimal integer string=w3319:string)  [unwired: 1 in]
                        n2270 = Search/Split String(string=w3323, search string/char (-)="_(" ("regular expression")) -> (substring before match=w3321:string)  [unwired: 1 in, 2 out]
                        n2271 = Concatenate Strings(w3321, "_(" ("regular expression"), w3319, ")" ("regular expression")) -> (w3317:string)
                        n2272 = local write "FILE"(w3317) -> ()
                      }
                    }
                  }
                  frame #1 {
                    w3326 = 0.0
                    w3339 = cluster{"y":dbl, dbl, "y":dbl}[] [] ("History Data")
                    w3340 = FALSE ("Heater Button")
                    (unwired) ")!" ("string")
                    (unwired) ")" ("string")
                    w3338 = dbl[] [] ("History Data")
                    w3344 = "\r"
                    # "C:\\WinDucom\\Data\\"
                    # "C:\\LAB-IQ-NXT\\data"
                    n2273 = local write "Humidity ( %RH )"(w3326) -> ()
                    n2274 = local write "Frequency ( Hz )"(w3326) -> ()
                    n2275 = local write "Stroke 3"(w3326) -> ()
                    n2276 = local write "speedop"(0.0 ("PIDclk 2")) -> ()
                    n2277 = local write "Set Temp 2"(65.0 ("Set Temp 2")) -> ()
                    n2278 = local write "AIR TEMP"(w3326) -> ()
                    n2279 = local write "clk"(0.0 ("clk")) -> ()
                    n2280 = local write "Stroke 4"(w3326) -> ()
                    n2281 = local write "COF 2"(w3326) -> ()
                    n2282 = local write "TEMP"(w3326) -> ()
                    n2283 = local write "ecr 3"(w3326) -> ()
                    n2284 = local write "FF 3"(w3326) -> ()
                    n2285 = local write "FF 2"(w3326) -> ()
                    n2286 = property on="Humidity ( %RH )" class="WFChart (strict)"("History Data"=w3338) -> ()  [unwired: 2 in, 2 out]
                    n2287 = property on="Coefficient of Friction" class="WFChart (strict)"("History Data"=w3338) -> ()  [unwired: 2 in, 2 out]
                    n2288 = property on="Coefficient of Friction" class="WFChart (strict)"("History Data"=w3338) -> ()  [unwired: 2 in, 2 out]
                    n2289 = property on="Frictional Force ( N )" class="WFChart (strict)"("History Data"=w3338) -> ()  [unwired: 2 in, 2 out]
                    n2290 = property on="Electrical Contact Resistance ( % )" class="WFChart (strict)"("History Data"=w3338) -> ()  [unwired: 2 in, 2 out]
                    n2291 = property on="Electrical Contact Resistance ( % )" class="WFChart (strict)"("History Data"=w3338) -> ()  [unwired: 2 in, 2 out]
                    n2292 = property on="Temperature ( Deg C )" class="WFChart (strict)"("History Data"=w3338) -> ()  [unwired: 2 in, 2 out]
                    n2293 = property on="Frictional Force ( N )" class="WFChart (strict)"("History Data"=w3338) -> ()  [unwired: 2 in, 2 out]
                    n2294 = property on="Coefficient of Friction" class="WFChart (strict)"("History Data"=w3338) -> ()  [unwired: 2 in, 2 out]
                    n2295 = property on="Frictional Force ( N )" class="WFChart (strict)"("History Data"=w3338) -> ()  [unwired: 2 in, 2 out]
                    n2296 = property on="Electrical Contact Resistance ( % )" class="WFChart (strict)"("History Data"=w3338) -> ()  [unwired: 2 in, 2 out]
                    n2297 = property on="Temperature ( Deg C )" class="WFChart (strict)"("History Data"=w3338) -> ()  [unwired: 2 in, 2 out]
                    n2298 = property on="Humidity ( %RH )" class="WFChart (strict)"("History Data"=w3338) -> ()  [unwired: 2 in, 2 out]
                    n2299 = property on="Stroke ( mm )" class="WFChart (strict)"("History Data"=w3339) -> ()  [unwired: 2 in, 2 out]
                    n2300 = property on="Stroke ( mm )" class="WFChart (strict)"("History Data"=w3339) -> ()  [unwired: 2 in, 2 out]
                    n2301 = local write "Humidity"(w3340) -> ()
                    n2302 = local write "Heater Button"(w3340) -> ()
                    n2303 = local read "FILE"() -> (w3334:string)
                    n2304 = disable-structure shown="Enabled" {
                      disable-tunnel: [w3378 _] -> w3325
                      frame Enabled {
                        n2305 = local read "NORMAL LOAD"() -> (w3378:dbl)
                      }
                      frame Disabled {
                      }
                    }
                    n2306 = call "file check.vi"("file name in"=w3334) -> ("error out"=w3337:errorcluster, "file name out"=w3331:string)  [unwired: 9 in]
                    n2307 = call "FILE PATH CREATION.vi"("error in"=w3337, "FILE NAME :"=w3331) -> ("FILE OUT"=w3330:path)  [unwired: 8 in, 1 out]
                    n2308 = Concatenate Strings(w3331, ".dgf" ("Substring")) -> (w3336:string)
                    n2309 = Concatenate Strings(w3331, ".duf" ("Substring")) -> (w3332:string)
                    n2310 = Multiply(x=w3325, y=1.0) -> (x*y=w3357:dbl)
                    n2311 = Build Path(base path=w3330, name or relative path=w3336) -> (appended path=w3329:path)
                    n2312 = Build Path(base path=w3330, name or relative path=w3332) -> (appended path=w3328:path)
                    n2313 = Number To Fractional String(number=w3357, width (-)=i16 5, precision (6)=i16 2) -> (F-format string=w3365:string)  [unwired: 1 in]
                    n2314 = local read "tested by"() -> (w3324:string)
                    n2315 = local read "Fuel Discription :"() -> (w3353:string)
                    n2316 = local read "Batch Ref Num :"() -> (w3342:string)
                    n2317 = Get Date/Time String(date format (0)=enum16{"short", "long", "abbreviated"}."short") -> (date string=w3376:string, time string=w3373:string)  [unwired: 2 in]
                    n2318 = local read "Remarks :"() -> (w3352:string)
                    n2319 = Concatenate Strings("Load :- " ("Substring"), w3365, " grams ," ("Substring")) -> (w3364:string)
                    n2320 = local read "String 41"() -> (w3345:string)
                    n2321 = Concatenate Strings(w3353) -> (w3354:string)
                    n2322 = Concatenate Strings(w3342) -> (w3341:string)
                    n2323 = Concatenate Strings(w3324) -> (w3348:string)
                    n2324 = Concatenate Strings("(" ("Substring"), w3376, ")" ("Substring"), w3373) -> (w3347:string)
                    "concatenated string" <- w3347
                    n2325 = Concatenate Strings(w3352, "," ("string")) -> (w3351:string)
                    n2326 = Concatenate Strings("  TIME;      COF;       STROKE;     AIR TEMP;  TEMP;  HUMIDITY;  ECR; PID-OUT; FREQUENCY" ("Substring"), "\r") -> (w3360:string)
                    n2327 = Concatenate Strings(w3345, w3344, "Fuel Discription :-" ("Substring"), w3354, w3344, w3364, w3344, "Batch Ref Num :-" ("Substring"), w3341, w3344, " Remarks :- " ("Substring"), w3351, w3344, " Date :- " ("Substring"), w3347, w3344, "Tested By :-" ("Substring"), w3348) -> (w3358:string)
                    "REMARKS" <- w3358
                    n2328 = call <vilib>:"Write Characters To File.vi"("append to file? (new file:F)"=FALSE, "character string"=w3360, "file path (dialog if empty)"=w3329) -> ()  [unwired: 2 in, 1 out]
                    n2329 = call <vilib>:"Write Characters To File.vi"("append to file? (new file:F)"=FALSE, "character string"=w3358, "file path (dialog if empty)"=w3328) -> ()  [unwired: 2 in, 1 out]
                  }
                  frame #2 {
                    n2330 = local write "Cycles elapsed"(0 ("Cycles elapsed")) -> ()
                    n2331 = local write "cyclecount"(0 ("cyclecount")) -> ()
                    n2332 = local write "Save & Continue"(FALSE ("OK")) -> ()
                    n2333 = local write "autostrtflg"(TRUE ("autostrtflg")) -> ()
                    n2334 = local write "Save"(FALSE ("Save")) -> ()
                    n2335 = Get Date/Time In Seconds() -> (seconds since 1Jan1904=w3383:timestamp)
                    n2336 = To Double Precision Float(number=w3383) -> (double precision float=w3382:dbl)
                    n2337 = local write "acq timer"(w3382) -> ()
                    n2338 = One Button Dialog(message="Please ensure sample is mounted properly and machine is ready in all aspects for testing !", button name ("OK")="Ok") -> ()  [unwired: 1 out]
                  }
                  frame #3 {
                    n2339 = stacked-sequence {
                      frame #0 {
                        n2340 = local write "Main Dashboard Buttons"(T1."Dashboard" ("Main Dashboard Buttons")) -> ()
                        n2341 = local write "Main Tab"(T2."Acquire" ("Main Tab")) -> ()
                      }
                      frame #1 {
                        n2342 = local write "EVENT LOG"("" ("EVENT LOG")) -> ()
                      }
                      frame #2 {
                        n2343 = Wait (ms)(milliseconds to wait=u32 50) -> ()  [unwired: 1 out]
                      }
                      frame #3 {
                        n2344 = disable-structure shown="Disabled" {
                          frame Disabled {
                            n2345 = local read "EVENT LOG"() -> (w3395:string)
                            n2346 = call "Event Log.vi"("Content"="Test Details", "EVENT LOG"=w3395) -> ("EVENT LOG"=w3394:string)  [unwired: 8 in, 1 out]
                            n2347 = local write "EVENT LOG"(w3394) -> ()
                          }
                          frame Enabled {
                          }
                        }
                      }
                      frame #4 {
                        n2348 = Wait (ms)(milliseconds to wait=u32 50) -> ()  [unwired: 1 out]
                      }
                      frame #5 {
                        n2349 = local read "FILE"() -> (w3397:string)
                        n2350 = Concatenate Strings("File Name :" ("Content"), w3397) -> (w3398:string)
                        n2351 = local read "EVENT LOG"() -> (w3401:string)
                        n2352 = call "Event Log.vi"("Content"=w3398, "EVENT LOG"=w3401) -> ("EVENT LOG"=w3400:string)  [unwired: 8 in, 1 out]
                        n2353 = local write "EVENT LOG"(w3400) -> ()
                      }
                      frame #6 {
                        n2354 = Wait (ms)(milliseconds to wait=u32 50) -> ()  [unwired: 1 out]
                      }
                      frame #7 {
                        n2355 = local read "Batch Ref Num :"() -> (w3403:string)
                        n2356 = Concatenate Strings("Batch Ref No :" ("Content"), w3403) -> (w3404:string)
                        n2357 = local read "EVENT LOG"() -> (w3407:string)
                        n2358 = call "Event Log.vi"("Content"=w3404, "EVENT LOG"=w3407) -> ("EVENT LOG"=w3406:string)  [unwired: 8 in, 1 out]
                        n2359 = local write "EVENT LOG"(w3406) -> ()
                      }
                      frame #8 {
                        n2360 = Wait (ms)(milliseconds to wait=u32 50) -> ()  [unwired: 1 out]
                      }
                      frame #9 {
                        n2361 = local read "tested by"() -> (w3409:string)
                        n2362 = Concatenate Strings("Tested By :" ("Content"), w3409) -> (w3410:string)
                        n2363 = local read "EVENT LOG"() -> (w3413:string)
                        n2364 = call "Event Log.vi"("Content"=w3410, "EVENT LOG"=w3413) -> ("EVENT LOG"=w3412:string)  [unwired: 8 in, 1 out]
                        n2365 = local write "EVENT LOG"(w3412) -> ()
                      }
                      frame #10 {
                        n2366 = Wait (ms)(milliseconds to wait=u32 50) -> ()  [unwired: 1 out]
                      }
                      frame #11 {
                        n2367 = local read "TEST STANDARD"() -> (w3416:T3)
                        n2368 = case shown="\"ASTM D6079\", Default" w3416 {
                          tunnel: ["ASTM D6079" "ISO 12156" "CEC F-096-A-06" "Custom"] -> w3415
                          frame "ASTM D6079", Default {
                          }
                          frame "ISO 12156" {
                          }
                          frame "CEC F-096-A-06" {
                          }
                          frame "Custom" {
                          }
                        }
                        n2369 = Concatenate Strings("Test Standard :" ("Content"), w3415) -> (w3417:string)
                        n2370 = local read "EVENT LOG"() -> (w3420:string)
                        n2371 = call "Event Log.vi"("Content"=w3417, "EVENT LOG"=w3420) -> ("EVENT LOG"=w3419:string)  [unwired: 8 in, 1 out]
                        n2372 = local write "EVENT LOG"(w3419) -> ()
                      }
                      frame #12 {
                        n2373 = Wait (ms)(milliseconds to wait=u32 50) -> ()  [unwired: 1 out]
                      }
                      frame #13 {
                        n2374 = local read "Fuel Discription :"() -> (w3426:string)
                        n2375 = Concatenate Strings("Fuel Description :" ("Content"), w3426) -> (w3427:string)
                        n2376 = local read "EVENT LOG"() -> (w3430:string)
                        n2377 = call "Event Log.vi"("Content"=w3427, "EVENT LOG"=w3430) -> ("EVENT LOG"=w3429:string)  [unwired: 8 in, 1 out]
                        n2378 = local write "EVENT LOG"(w3429) -> ()
                      }
                      frame #14 {
                        n2379 = Wait (ms)(milliseconds to wait=u32 50) -> ()  [unwired: 1 out]
                      }
                      frame #15 {
                        n2380 = local read "Remarks :"() -> (w3432:string)
                        n2381 = Concatenate Strings("Remarks :" ("Content"), w3432) -> (w3433:string)
                        n2382 = local read "EVENT LOG"() -> (w3436:string)
                        n2383 = call "Event Log.vi"("Content"=w3433, "EVENT LOG"=w3436) -> ("EVENT LOG"=w3435:string)  [unwired: 8 in, 1 out]
                        n2384 = local write "EVENT LOG"(w3435) -> ()
                      }
                      frame #16 {
                        n2385 = Wait (ms)(milliseconds to wait=u32 50) -> ()  [unwired: 1 out]
                      }
                      frame #17 {
                        n2386 = local read "USER ID"() -> (w3438:string)
                        n2387 = Concatenate Strings("Operator ID :" ("Content"), w3438) -> (w3440:string)
                        n2388 = local read "EVENT LOG"() -> (w3442:string)
                        n2389 = call "Event Log.vi"("Content"=w3440, "EVENT LOG"=w3442) -> ("EVENT LOG"=w3441:string)  [unwired: 8 in, 1 out]
                        n2390 = local write "EVENT LOG"(w3441) -> ()
                      }
                      frame #18 {
                        n2391 = Wait (ms)(milliseconds to wait=u32 50) -> ()  [unwired: 1 out]
                      }
                      frame #19 {
                        n2392 = disable-structure shown="Disabled" {
                          frame Disabled {
                            n2393 = local read "EVENT LOG"() -> (w3446:string)
                            n2394 = call "Event Log.vi"("Content"="Test Parameter", "EVENT LOG"=w3446) -> ("EVENT LOG"=w3445:string)  [unwired: 8 in, 1 out]
                            n2395 = local write "EVENT LOG"(w3445) -> ()
                          }
                          frame Enabled {
                          }
                        }
                      }
                      frame #20 {
                        n2396 = Wait (ms)(milliseconds to wait=u32 50) -> ()  [unwired: 1 out]
                      }
                      frame #21 {
                        n2397 = local read "Set Hz"() -> (w3450:dbl)
                        n2398 = Number To Fractional String(number=w3450, precision (6)=i16 2) -> (F-format string=w3449:string)  [unwired: 2 in]
                        n2399 = Concatenate Strings("Set Frequency [Hz] :" ("Content"), w3449) -> (w3452:string)
                        n2400 = local read "EVENT LOG"() -> (w3454:string)
                        n2401 = call "Event Log.vi"("Content"=w3452, "EVENT LOG"=w3454) -> ("EVENT LOG"=w3453:string)  [unwired: 8 in, 1 out]
                        n2402 = local write "EVENT LOG"(w3453) -> ()
                      }
                      frame #22 {
                        n2403 = Wait (ms)(milliseconds to wait=u32 50) -> ()  [unwired: 1 out]
                      }
                      frame #23 {
                        n2404 = local read "NORMAL LOAD"() -> (w3457:dbl)
                        n2405 = Number To Fractional String(number=w3457, precision (6)=i16 2) -> (F-format string=w3458:string)  [unwired: 2 in]
                        n2406 = Concatenate Strings("Applied Load [grams] :" ("Content"), w3458) -> (w3460:string)
                        n2407 = local read "EVENT LOG"() -> (w3462:string)
                        n2408 = call "Event Log.vi"("Content"=w3460, "EVENT LOG"=w3462) -> ("EVENT LOG"=w3461:string)  [unwired: 8 in, 1 out]
                        n2409 = local write "EVENT LOG"(w3461) -> ()
                      }
                      frame #24 {
                        n2410 = Wait (ms)(milliseconds to wait=u32 50) -> ()  [unwired: 1 out]
                      }
                      frame #25 {
